vi "Auto Config Monitored Channels.vi"(7 "Protection Type":T2=enum."LP_CRC8", 8 "error in (no error)":errorcluster, 11 "Protection Value Ref":T1 format="%.0x") -> (0 "error out":errorcluster, 3 "Protection Value Ref Out":T1=18446744073709551615 format="%.0x")   [LabVIEW 2023, in "Protection and Counter Support System Explorer.lvlib"]
uses:
  Protection and Counter Support System Explorer.lvlib
  <vilib>/NI VeriStand/Custom Device API/Custom Device Item Ref.ctl
  Shared/Types/Protection Type.ctl
  Types/Protection Signal Settings.ctl
  Types/Protection Signal Linked Channel.ctl
  Addon/Addon Shared/SubVIs/GUID Lookup.vi
  <vilib>/NI VeriStand/Custom Device API/Custom Device API.lvlib
  Shared/Protection and Counter Support Shared.lvlib
  Addon/Addon Shared/Protection and Counter Addon Shared.lvlib
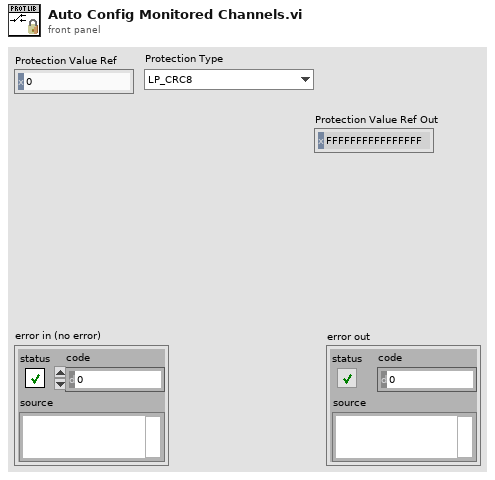
[diagram p1: front panel]
types:
  T1 = typedef "Custom Device API.lvlib/Custom Device Item Ref.ctl" = u64
  T2 = typedef "Protection and Counter Support Shared.lvlib/Protection Type.ctl" = enum16{"Arb ID + Bytes Checksum with Inversion", "Arb ID + Bytes CRC with Inversion", "Reversed Raw Signal Checksum with Inversion", "Concatenated Two's Compliment", "LP_CRC8", "LP_Checksum", "LP_CRC8_MRS"}
  T3 = typedef "Protection and Counter Support System Explorer.lvlib/Protection Signal Settings.ctl" = cluster{"Input Channels":T4[], "Protection Type":T2}
  T4 = typedef "Protection and Counter Support System Explorer.lvlib/Protection Signal Linked Channel.ctl" = cluster{"Node Ref":T1}
  T5 = typedef "Custom Device API.lvlib/Custom Device Item Info.ctl" = cluster{"Name":string, "Is Channel":bool, "GUID":string, "Is Waveform":bool}
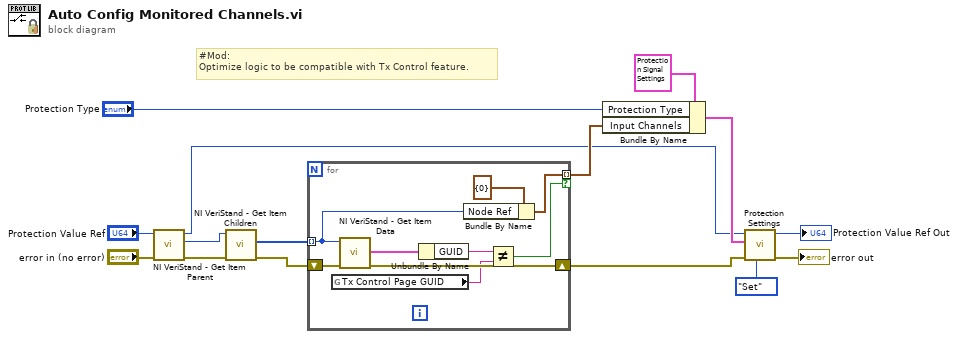
[diagram p0: block diagram]
diagram:
  # "#Mod:\nOptimize logic to be compatible with Tx Control feature."
  n1 = call <vilib>:"NI VeriStand - Get Item Parent.vi"("error in (no error)"="error in (no error)", "Item Ref in"="Protection Value Ref") -> ("error out"=w1:errorcluster, "Parent Ref"=w3:T1, "Item Ref out"=w2:T1)  [unwired: 6 in, 1 out]
  n2 = call <vilib>:"NI VeriStand - Get Item Children.vi"("error in (no error)"=w1, "Item Ref in"=w3) -> ("error out"=w5:errorcluster, "Child Refs"=w7:T1[])  [unwired: 6 in, 2 out]
  n3 = for {
    tunnel: w7 -> [w20] mode=indexing
    tunnel: [w21] -> w6 mode=indexing if=w16
    shift-right: [w23] -> w4
    shift-left: w5 -> [w24]
    n4 = global read "GUID Lookup.vi" "Tx Control Page GUID"() -> (w17:string)
    n5 = call <vilib>:"NI VeriStand - Get Item Data.vi"("error in (no error)"=w24, "Item Ref in"=w20) -> ("error out"=w23:errorcluster, "Item Info"=w19:T5)  [unwired: 6 in, 2 out]
    n6 = Unbundle By Name(w19) -> ("GUID"=w18:string)
    n7 = Bundle By Name(cluster=T4 {"Node Ref"=0} ("MonitoredChannelSettings"), "Node Ref"=w20) -> (w21:T4)
    n8 = Not Equal?(x=w18, y=w17) -> (x != y?=w16:bool)
  }
  n9 = Bundle By Name(cluster=T3 {"Input Channels"=[], "Protection Type"=enum."Arb ID + Bytes Checksum with Inversion"} ("Selected Channels"), "Protection Type"="Protection Type", "Input Channels"=w6) -> (w8:T3)
  n10 = call "Protection Settings.vi"("Action"=enum8{"Get", "Set"}."Set", "error in"=w4, "Selected Channels"=w8, "Parent Ref"=w2) -> ("error out"=→"error out":errorcluster, "Parent Ref Out"=→"Protection Value Ref Out":T1)  [unwired: 5 in, 1 out]
